vi "Read metadata from tiff string.vi"(8 "error in":errorcluster, 9 "DirEntries":T1[](array[typedef]), 10 "Tiff image stack":string, 11 "Tiff image stack":refnum<file>) -> (0 "error out":errorcluster, 1 "Metadata string":string, 2 "Tag exists?":bool, 3 "Tiff image stack dup":refnum<file>)   [LabVIEW 2015, in "Tiff reader.lvlib"]
doc: "This .vi reads metadata from the tiff file (represented as a string or file refnum)."
uses:
  Tiff reader.lvlib
  FieldTypes.ctl
  IFD Entry.ctl
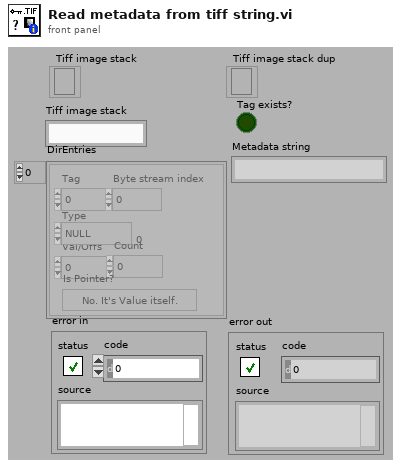
[diagram p1: front panel]
types:
  T1 = typedef "Tiff reader.lvlib/IFD Entry.ctl" = cluster{"Tag":u16, "Type":T2, "Count":u32, "Val/Offs":u32, "Is Pointer?":bool, "Byte stream index":i32}
  T2 = typedef "Tiff reader.lvlib/FieldTypes.ctl" = enum16{"NULL", "U8", "ASCII7", "U16", "U32", "RATIONAL", "SByte(I8)", "Undef(8Bit)", "I16", "I32", "SRat(4B:4B)", "SGL(4Byte)", "DBL(8Byte)"}
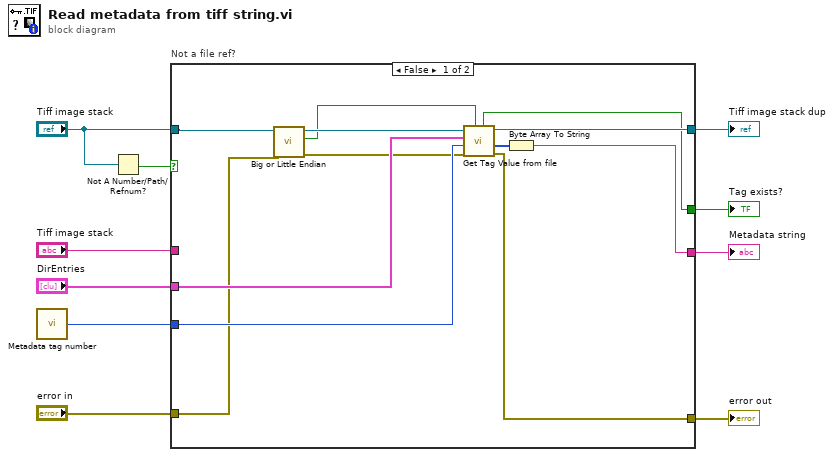
[diagram p0: block diagram]
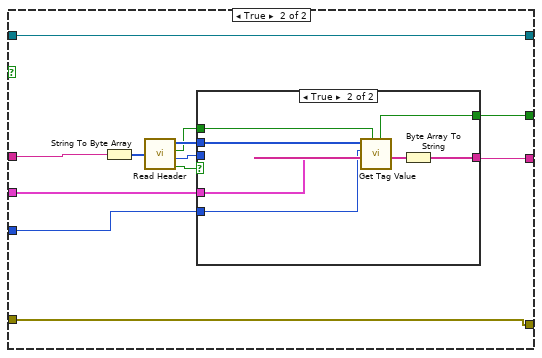
[diagram p2: hidden frame]
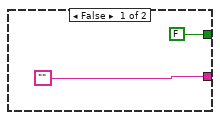
[diagram p3: hidden frame]
diagram:
  n1 = call "Metadata tag number.vi"() -> ("Tag to store\nmetadata in\n(ImageID tag)"=w7:u16)
  n2 = Not A Number/Path/Refnum?(number/path/refnum="Tiff image stack") -> (NaN/Path/Refnum?=w6:bool)
  n3 = case "Not a file ref?" shown="False" w6 {
    tunnel: "Tiff image stack" -> [_ w33]
    tunnel: [w19 w28] -> w9
    tunnel: "DirEntries" -> [w16 w27]
    tunnel: w7 -> [w21 w26]
    tunnel: "Tiff image stack" -> [w14 w25]
    tunnel: [w22 w25] -> w4
    tunnel: [w18 w24] -> w3
    tunnel: "error in" -> [w13 w24]
    tunnel: [w17 w23] -> w1
    frame False {
      n4 = call "Big or Little Endian.vi"("error in"=w13, "File"=w14) -> ("error out"=w12:errorcluster, "Litt/BigEnd"=w11:bool, "File out"=w15:refnum<file>)  [unwired: 7 out]
      n5 = call "Get Tag Value from file.vi"("Litt/BigEnd"=w11, "error in"=w12, "Tag Code"=w21, "DirEntries"=w16, "File"=w15) -> ("error out"=w18:errorcluster, "Multiple Values"=w20:u64[], "File"=w22:refnum<file>, "Tag exists?"=w17:bool)  [unwired: 3 out]
      n6 = Byte Array To String(unsigned byte array=w20) -> (string=w19:string)
    }
    frame True {
      n7 = String To Byte Array(string=w33) -> (unsigned byte array=w34:u8[])
      n8 = call "Read Header.vi"("TIFF Data in"=w34) -> ("TIFF Data out"=w31:u8[], "Litt/BigEnd"=w30:bool, "ImFileDirectOffs"=w29:u32, "IsTIFF?"=w32:bool)
      n9 = case shown="True" w32 {
        tunnel: w31 -> [_ w38]
        tunnel: w30 -> [_ w43]
        tunnel: w29 -> [_ _]
        tunnel: w26 -> [_ w42]
        tunnel: ["" w40] -> w28
        tunnel: w27 -> [_ w37]
        tunnel: [FALSE ("Tag exists?") w39] -> w23
        frame False {
        }
        frame True {
          n10 = call "Get Tag Value.vi"("Litt/BigEnd"=w43, "DirEntries"=w37, "Tag Code"=w42, "Image Data in"=w38) -> ("Multiple Values"=w41:u64[], "Tag exists?"=w39:bool)  [unwired: 4 out]
          n11 = Byte Array To String(unsigned byte array=w41) -> (string=w40:string)
        }
      }
    }
  }
  "Metadata string" <- w9
  "Tiff image stack dup" <- w4
  "error out" <- w3
  "Tag exists?" <- w1
